vi "Create.vi"(5 "ErrorCode In":refnum<class "ErrorCode.lvclass">, 8 "error in (no error)":errorcluster, 10 "Expected":i32) -> (0 "error out":errorcluster, 3 "ErrorCode":refnum<class "ErrorCode.lvclass">)   [LabVIEW 2019, in "Constraint.lvlib" / "ErrorCode.lvclass"]
uses:
  ErrorCode.lvclass
  ErrorCode.lvclass/ErrorCode.ctl
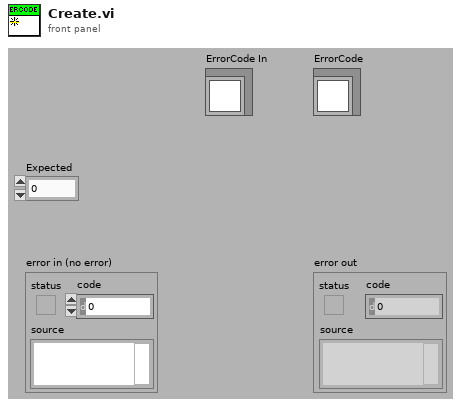
[diagram p1: front panel]
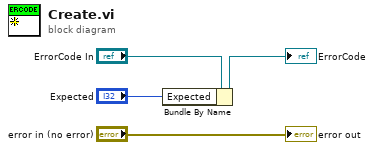
[diagram p0: block diagram]
diagram:
  n1 = Bundle By Name(cluster="ErrorCode In", "Expected"="Expected") -> (→"ErrorCode":refnum<class "ErrorCode.lvclass">)
  "error out" <- "error in (no error)"
